vi "Write (DBL).vi"(6 "Data":dbl[](array[numeric]), 8 "error in (no error)":errorcluster, 9 "Channel name":string, 10 "Group name":string, 11 "File in":refnum<class "File.lvclass">) -> (0 "error out":errorcluster, 1 "Channel name out":string, 2 "Group name out":string, 3 "File out":refnum<class "File.lvclass">)   [LabVIEW 2016, in "File.lvclass"]
uses:
  File.lvclass
  File.lvclass/File.ctl
  Read tdms stream.vi
  Write tdms stream.vi
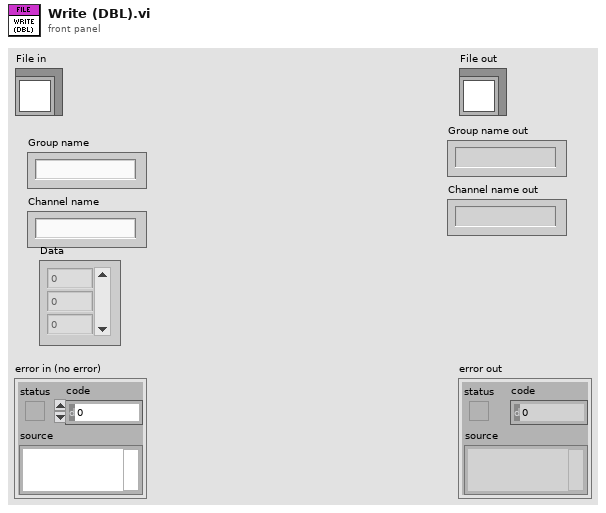
[diagram p1: front panel]
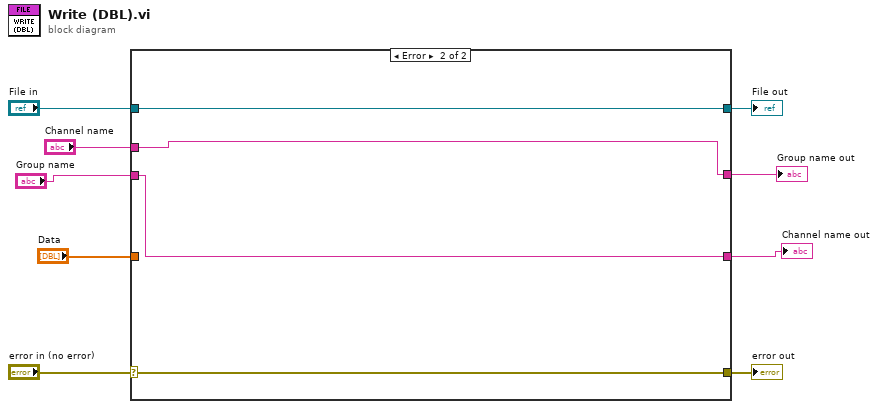
[diagram p0: block diagram]
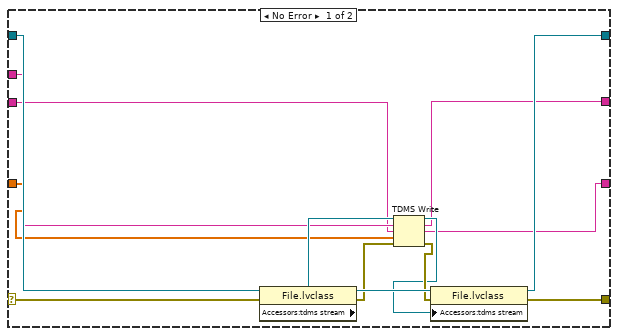
[diagram p2: hidden frame]
diagram:
  n1 = case shown="Error" "error in (no error)" {
    selector: "error in (no error)" -> [w23 w27]
    tunnel: [w21 w27] -> w8
    tunnel: [w19 w26] -> w6
    tunnel: "File in" -> [w22 w26]
    tunnel: "Group name" -> [w13 w24]
    tunnel: "Data" -> [w12 _]
    tunnel: "Channel name" -> [w14 w25]
    tunnel: [w11 w25] -> w2
    tunnel: [w10 w24] -> w1
    frame No Error {
      n2 = property class="File.lvclass"(reference=w22, error in=w23) -> (reference out=w20:refnum<class "File.lvclass">, error out=w18:errorcluster, "Accessors:tdms stream"=w16:refnum<k34>)
      n3 = TDMS Write(0:w16, 5:w14, 7:w13, 9:w12, 11:w18) -> (4:w15:refnum<k34>, 6:w11:string, 8:w10:string, 15:w17:errorcluster)  [unwired: 1 in]
      n4 = property class="File.lvclass"(reference=w20, error in=w17, "Accessors:tdms stream"=w15) -> (reference out=w19:refnum<class "File.lvclass">, error out=w21:errorcluster)
    }
    frame Error {
    }
  }
  "error out" <- w8
  "File out" <- w6
  "Channel name out" <- w1
  "Group name out" <- w2
